vi "Call Subpanel VI.vi"(8 "error in (no error)":errorcluster, 10 "VI Refnum":refnum<vi>, 11 "UserPwd DB Configuration in":refnum<class "UserPwd DB Configuration.lvclass">) -> (0 "error out":errorcluster, 3 "UserPwd DB Configuration out":refnum<class "UserPwd DB Configuration.lvclass">)   [LabVIEW 2016, in "UserPwd DB.lvlib" / "UserPwd DB Configuration.lvclass"]
uses:
  <userlib>/Common Components/UserPwd DB/UserPwd DB Config/UserPwd DB Configuration.lvclass
  <userlib>/Configuration Dialog Actor/Configuration.lvclass
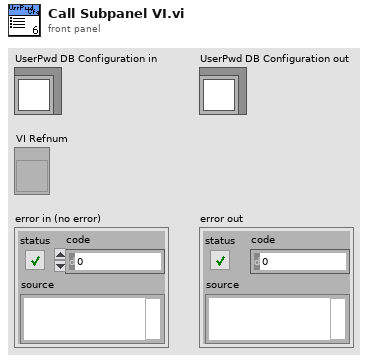
[diagram p1: front panel]
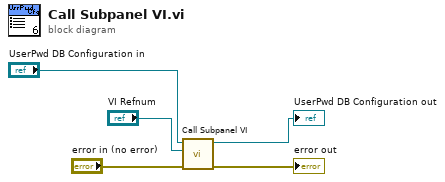
[diagram p0: block diagram]
diagram:
  n1 = call-parent "Call Subpanel VI.vi"("error in (no error)"="error in (no error)", "VI Refnum"="VI Refnum", "Configuration in"="UserPwd DB Configuration in") -> ("error out"=→"error out":errorcluster, "Configuration out"=→"UserPwd DB Configuration out":refnum<class "UserPwd DB Configuration.lvclass">)  [unwired: 7 in]
